vi "MsgCfgParser.vi"(1 "search string":string, 2 "name or relative path":string, 3 "stripped path":path) -> (0 "Cluster Array":T1(array[cluster]))   [LabVIEW 2010]
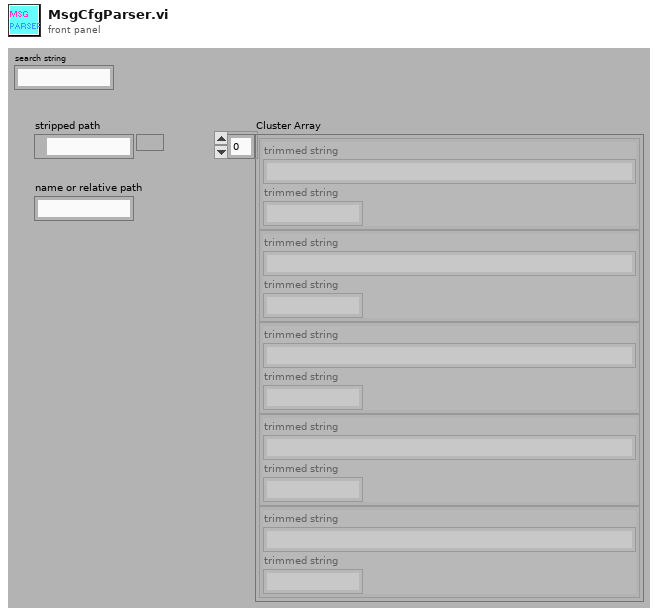
[diagram p1: front panel]
types:
  T1 = cluster{"trimmed string":string, "trimmed string":string}[]
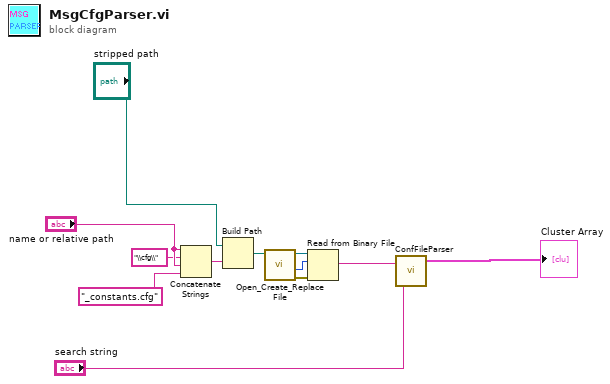
[diagram p0: block diagram]
diagram:
  n1 = Concatenate Strings("name or relative path", "\\cfg\\" ("string"), "name or relative path", "_constants.cfg" ("name or relative path")) -> (w2:string)
  n2 = Build Path(base path="stripped path", name or relative path=w2) -> (appended path=w4:path)
  n3 = call <vilib>:"Open_Create_Replace File.vi"("file path"=w4) -> ("error out"=w5:errorcluster, "file size (bytes)"=w6:i32, "refnum"=w7:refnum<file>)  [unwired: 7 in, 1 out]
  n4 = Read from Binary File(8:w5, 10:w6, 11:w7) -> (2:w10:string)  [unwired: 3 in, 3 out]
  n5 = call "ConfFileParser.vi"("TEXT"=w10, "search string"="search string") -> ("Cluster Array"=→"Cluster Array":T1)  [unwired: 2 out]
